vi "DQMH_API_Script New Event.vi"(0 "LibraryPath":path, 1 "Project":refnum<vi>, 2 "Add Tester Button":bool, 3 "Event Description":string, 4 "Open Main and Tester? (F)":bool, 5 "Existing Argument Path":path, 7 "Event Name":string, 9 "Event Type":T1, 11 "Custom Enqueue VI":path, 14 "Round Trip (Broadcast)":string) -> (15 "error out":errorcluster)   [LabVIEW 2016]
uses:
  project/Delacor/DQMH/_DQMH New Event/Event Type--enum.ctl
  project/Delacor/DQMH/_support/Scripting Identifiers--global.vi
  project/Delacor/DQMH/_DQMH New Event/DQMH New Event.lvlib
  project/Delacor/DQMH/_support/_DQMH Scripting Support.lvlib
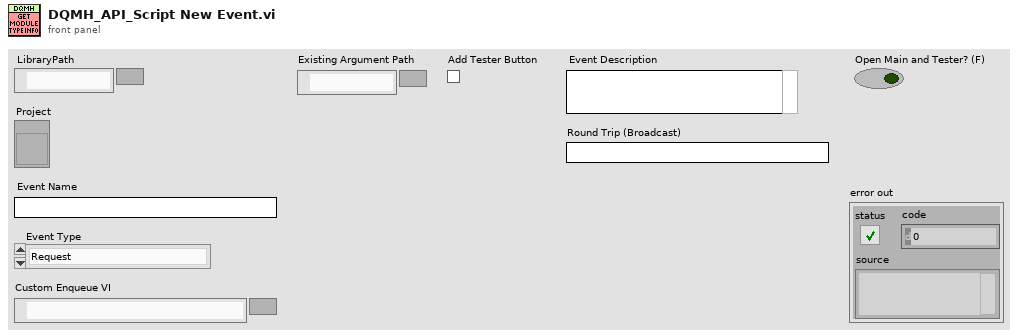
[diagram p1: front panel]
types:
  T1 = typedef "DQMH New Event.lvlib/Event Type--enum.ctl" = enum16{"Request", "Broadcast", "Request and Wait for Reply", "Round Trip"}
  T2 = typedef "DQMH New Event.lvlib/Module Info--cluster.ctl" = cluster{"Name":string, "Library":refnum<vi>, "Library Owning App":refnum<vi>, "Library Owning Folder":path, "Module Type":T3, "Public API Requests Folder":refnum<vi>, "Public API Requests Arguments Folder":refnum<vi>, "Broadcasts Folder":refnum<vi>, "Broadcasts Arguments Folder":refnum<vi>, "Obtain Broadcast Events VI":refnum<vi>, "Destroy Broadcast Events VI":refnum<vi>, "Obtain Request Events VI":refnum<vi>, "Destroy Request Events VI":refnum<vi>, "Request Events Cluster CTL":refnum<vi>, "Broadcast Events Cluster CTL":refnum<vi>, "Module Timeout VI":refnum<vi>, "Module Name VI":refnum<vi>, "Status Updated VI":refnum<vi>, "Module Not Running Error Constant VI":refnum<vi>}
  T3 = typedef "DQMH New Event.lvlib/Module Type--enum.ctl" = enum16{"Singleton", "Cloneable"}
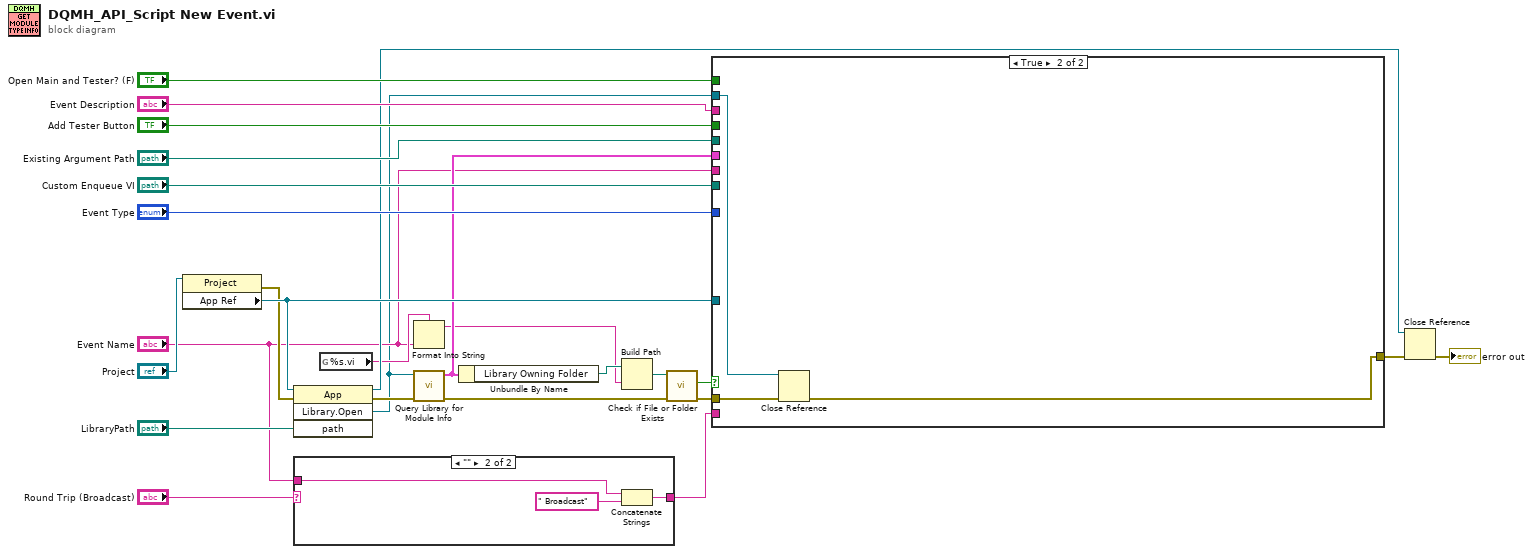
[diagram p0: block diagram]
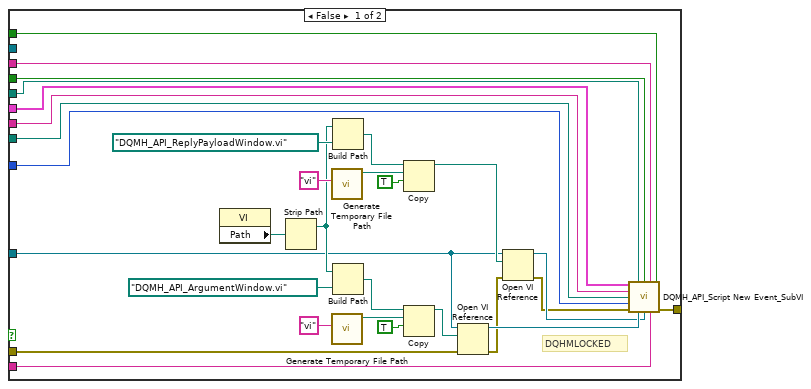
[diagram p2: hidden frame]
diagram:
  n1 = property class="Project"(reference="Project") -> (error out=w15:errorcluster, "App Ref"=w17:refnum<vi>)  [unwired: 1 in, 1 out]
  n2 = invoke class="App" method="Library.Open"(reference=w17, error in=w15, "path"="LibraryPath") -> (reference out=w14:refnum<vi>, error out=w5:errorcluster, "Open Library"=w1:refnum<vi>)  [unwired: 1 in, 1 out]
  n3 = case shown="\"\"" "Round Trip (Broadcast)" {
    selector: "Round Trip (Broadcast)" -> [w27 _]
    tunnel: "Event Name" -> [_ w30]
    tunnel: [w27 w28] -> w19
    frame Default {
    }
    frame "" {
      n4 = Concatenate Strings(w30, " Broadcast" ("format string")) -> (w28:string)
    }
  }
  n5 = global read "Scripting Identifiers--global.vi" "%s.vi"() -> (w10:string)
  n6 = Format Into String(format string=w10, "Event Name") -> (resulting string=w7:string)  [unwired: 2 in, 1 out]
  n7 = call "Query Library for Module Info.vi"("error in (no error)"=w5, "Library"=w1) -> ("error out"=w4:errorcluster, "Module Info"=w11:T2)  [unwired: 5 in, 3 out]
  n8 = Unbundle By Name(w11) -> ("Library Owning Folder"=w9:path)
  n9 = Build Path(base path=w9, name or relative path=w7) -> (appended path=w6:path)
  n10 = call <vilib>:"Check if File or Folder Exists.vi"("error in (no error)"=w4, "path"=w6) -> ("error out"=w3:errorcluster, "file or folder exists?"=w2:bool)  [unwired: 7 in, 1 out]
  n11 = case shown="True" w2 {
    tunnel: "Event Description" -> [w60 _]
    tunnel: "Existing Argument Path" -> [w59 _]
    tunnel: "Add Tester Button" -> [w58 _]
    tunnel: "Event Type" -> [w57 _]
    tunnel: "Open Main and Tester? (F)" -> [w56 _]
    tunnel: "Custom Enqueue VI" -> [w55 _]
    tunnel: w19 -> [w38 _]
    tunnel: w17 -> [w37 _]
    tunnel: [w35 w61] -> w12
    tunnel: w11 -> [w34 _]
    tunnel: "Event Name" -> [w33 _]
    tunnel: w3 -> [w31 w62]
    tunnel: w1 -> [_ w63]
    frame False {
      # "DQHMLOCKED"
      n12 = property class="VI"() -> ("Path"=w53:path)  [unwired: 2 in, 2 out]
      n13 = Strip Path(path=w53) -> (stripped path=w40:path)  [unwired: 1 out]
      n14 = call <vilib>:"Generate Temporary File Path.vi"("Temporary File Extension (tmp)"="vi") -> ("Unique Temporary File Path"=w44:path)  [unwired: 9 in, 1 out]
      n15 = call <vilib>:"Generate Temporary File Path.vi"("Temporary File Extension (tmp)"="vi") -> ("Unique Temporary File Path"=w50:path)  [unwired: 9 in, 1 out]
      n16 = Build Path(base path=w40, name or relative path=path "DQMH_API_ReplyPayloadWindow.vi") -> (appended path=w43:path)
      n17 = Build Path(base path=w40, name or relative path=path "DQMH_API_ArgumentWindow.vi") -> (appended path=w51:path)
      n18 = Copy(9:TRUE ("overwrite (F)"), 10:w44, 11:w43) -> (3:w46:path)  [unwired: 2 in, 2 out]
      n19 = Copy(9:TRUE ("overwrite (F)"), 10:w50, 11:w51) -> (3:w48:path)  [unwired: 2 in, 2 out]
      n20 = Open VI Reference(application reference (local)=w37, vi path=w48, error in (no error)=w31) -> (vi reference=w47:refnum<vi>, error out=w36:errorcluster)  [unwired: 3 in]
      n21 = Open VI Reference(application reference (local)=w37, vi path=w46, error in (no error)=w36) -> (vi reference=w39:refnum<vi>, error out=w32:errorcluster)  [unwired: 3 in]
      n22 = call <resource>:"DQMH_API_Script New Event_SubVI.vi"("Module Info"=w34, "Existing Argument Path"=w59, "Add Tester Button"=w58, "Event Description"=w60, "Open Main and Tester? (T)"=w56, "Event Name"=w33, "Custom Enqueue VI"=w55, "Event Type"=w57, "error in (no error)"=w32, "Arguments VI"=w47, "Reply Payload VI"=w39, "Round Trip (Broadcast)"=w38) -> ("error out"=w35:errorcluster)  [unwired: 3 in]
    }
    frame True {
      n23 = Close Reference(reference=w63, error in (no error)=w62) -> (error out=w61:errorcluster)
    }
  }
  n24 = Close Reference(reference=w14, error in (no error)=w12) -> (error out=→"error out":errorcluster)
